vi "Snap 90 implementation.vi"(10 "YawWrap":dbl) -> (2 "Snap Goal":dbl=-90.0)   [LabVIEW 2018]
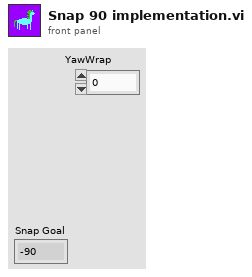
[diagram p1: front panel]
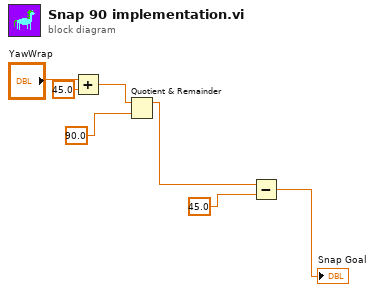
[diagram p0: block diagram]
diagram:
  n1 = Add(x="YawWrap", y=45.0) -> (x+y=w5:dbl)
  n2 = Quotient & Remainder(x=w5, y=90.0) -> (x-y*floor(x/y)=w3:dbl)  [unwired: 1 out]
  n3 = Subtract(x=w3, y=45.0) -> (x-y=→"Snap Goal":dbl)
